vi "S2C_VAR_NewSelection.vi"(7 "Action":enum16{"Add", "Delete"}(ring), 8 "Error In":errorcluster, 11 "Ref In":refnum<vi>) -> (0 "Error Out":errorcluster, 3 "Ref Out":refnum<vi>)   [LabVIEW 2015]
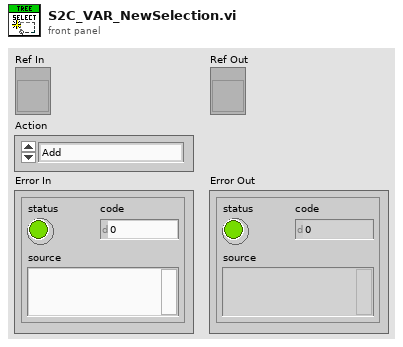
[diagram p1: front panel]
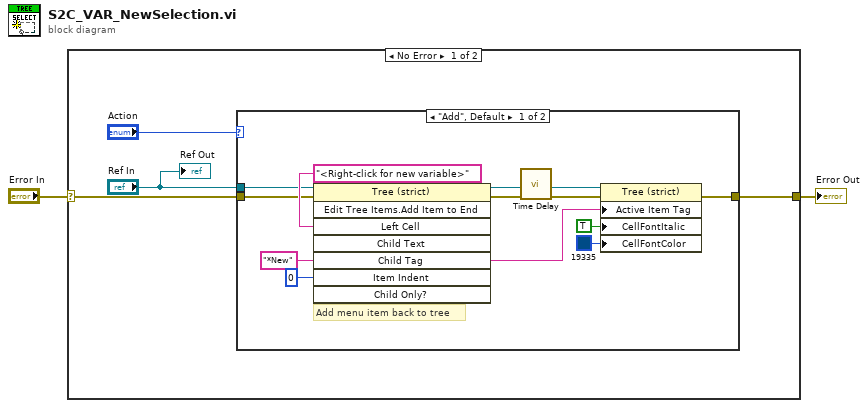
[diagram p0: block diagram]
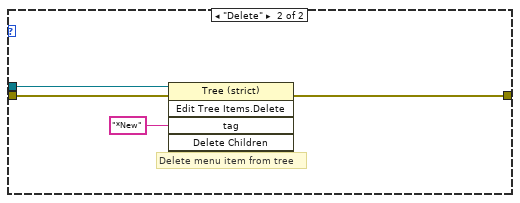
[diagram p2: hidden frame]
diagram:
  n1 = case shown="No Error" "Error In" {
    selector: "Error In" -> [w6 w22]
    tunnel: [w4 w22] -> w1
    frame No Error {
      n2 = case shown="\"Add\", Default" "Action" {
        tunnel: w6 -> [w15 w21]
        tunnel: [w11 w18] -> w4
        tunnel: "Ref In" -> [w14 w20]
        frame "Add", Default {
          w9 = "*New" ("Tag")
          # "Add menu item back to tree"
          n3 = invoke class="Tree (strict)" method="Edit Tree Items.Add Item to End"(reference=w14, error in=w15, "Left Cell"="<Right-click for new variable>" ("Name"), "Child Tag"=w9, "Item Indent"=0 ("New Item Indentation")) -> (reference out=w10:refnum<vi>, error out=w8:errorcluster)  [unwired: 3 in, 6 out]
          n4 = call "Time Delay"("error in (no error)"=w8) -> ("error out"=w7:errorcluster)  [unwired: 10 in]
          n5 = property class="Tree (strict)"(reference=w10, error in=w7, "Active Item Tag"=w9, "CellFontItalic"=TRUE ("Active Cell:Cell Font:Italic"), "CellFontColor"=u32 19335) -> (error out=w11:errorcluster)  [unwired: 1 out]
        }
        frame "Delete" {
          # "Delete menu item from tree"
          n6 = invoke class="Tree (strict)" method="Edit Tree Items.Delete"(reference=w20, error in=w21, "tag"="*New" ("Tag")) -> (error out=w18:errorcluster)  [unwired: 2 in, 4 out]
        }
      }
      "Ref Out" <- "Ref In"
    }
    frame Error {
    }
  }
  "Error Out" <- w1
